vi "37 Time Conversion (x64-2018).vi"(10 "CPU Time In":dbl format="%#.6f", 11 "Time In":string) -> (3 "Time Out":string)   [LabVIEW 2017]
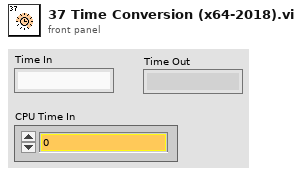
[diagram p1: front panel]
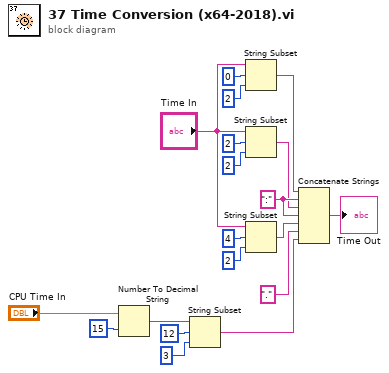
[diagram p0: block diagram]
diagram:
  w10 = ":"
  n1 = Number To Decimal String(number="CPU Time In", width (-)=15) -> (decimal integer string=w14:string)
  n2 = String Subset(string=w14, offset (0)=12, length (rest)=3) -> (substring=w18:string)
  n3 = String Subset(string="Time In", offset (0)=0, length (rest)=2) -> (substring=w8:string)
  n4 = String Subset(string="Time In", offset (0)=2, length (rest)=2) -> (substring=w9:string)
  n5 = String Subset(string="Time In", offset (0)=4, length (rest)=2) -> (substring=w11:string)
  n6 = Concatenate Strings(w8, w10, w9, w10, w11, ".", w18) -> (→"Time Out":string)
